vi "CALC_LIM_DATA.vi"(0 "VISA IN":refnum<visa-resource-name>, 1 "Data":string, 5 "error in":errorcluster, 7 "Channel":i32) -> (14 "VISA Out":refnum<visa-resource-name>, 19 "error out":errorcluster)   [LabVIEW 2018, in "PNA-X.lvlib"]
doc: "CALCulate<cnum>:LIMit:DATA <block> \n(Read-Write) Sets data for limit segments. \nSee Critical Note \nParameters \n<cnum> Channel number of the measurement. There must be a selected measurement \non that channel. If unspecified, <cnum> is set to 1. \n<block> Data for all limit segments in REAL,64 format. The following is the data \nformat for 1 segment: \nType,BegStim, EndStim, BegResp,EndResp \n1521\n\nType Type of limit segment. Choose from \n0 - Off \n1 - Max \n2 - Min \nBegStim Start of X-axis value (freq, power, time) \nEndStim End of X-axis value \nBegResp Y-axis value that corresponds with Start of X-axis value \nEndResp Y-axis value that corresponds with End of X-axis value \nExamples The following writes three max limit segments for a bandpass filter. \n\"CALC:LIM:DATA 1,3e5,4e9,-60,0,1,4e9,7.5e9,0,0,1,7.5e9,9e9,0,- \n30\" \nQuery Syntax CALCulate<cnum>:LIMit:DATA? \nReturn Type Depends on FORM:DATA - All 100 predefined limit segments are returned. \nDefault 100 limit segments - all values set to 0"
uses:
  PNA-X.lvlib
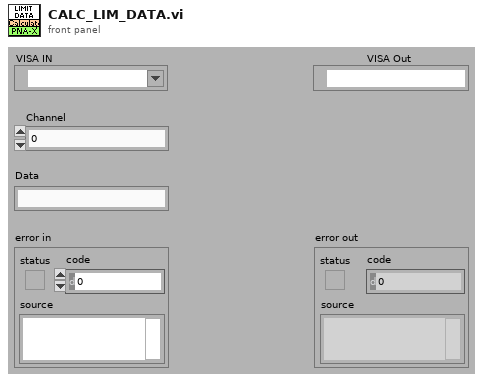
[diagram p1: front panel]
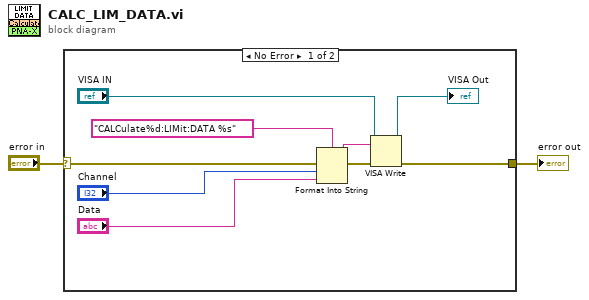
[diagram p0: block diagram]
diagram:
  n1 = case shown="No Error" "error in" {
    selector: "error in" -> [w11 w12]
    tunnel: [w6 w12] -> w1
    frame No Error {
      n2 = Format Into String(format string="CALCulate%d:LIMit:DATA %s" ("Cmdline"), error in=w11, "Channel", "Data") -> (resulting string=w9:string, error out=w10:errorcluster)  [unwired: 1 in]
      n3 = VISA Write(VISA resource name="VISA IN", write buffer=w9, error in (no error)=w10) -> (VISA resource name out=→"VISA Out":refnum<visa-resource-name>, error out=w6:errorcluster)  [unwired: 1 out]
    }
    frame Error {
    }
  }
  "error out" <- w1
